vi "File_Driver.vi"(0 "File_Path":path, 2 "Section":string, 5 "Data_In":string, 7 "Key":string, 11 "Error_In":errorcluster, 13 "File_Operation_Select":T1=enum."Close") -> (6 "Data_Out":string, 15 "Error_Out":errorcluster)   [LabVIEW 2021]
uses:
  <vilib>/Utility/config.llb/NI_LVConfig.lvlib
  <vilib>/Utility/config.llb/Read Key (String).vi
  <vilib>/Utility/config.llb/Config Data RefNum.ctl
  <vilib>/Utility/config.llb/Write Key (String).vi
  Controls/File_Operation_Select.ctl
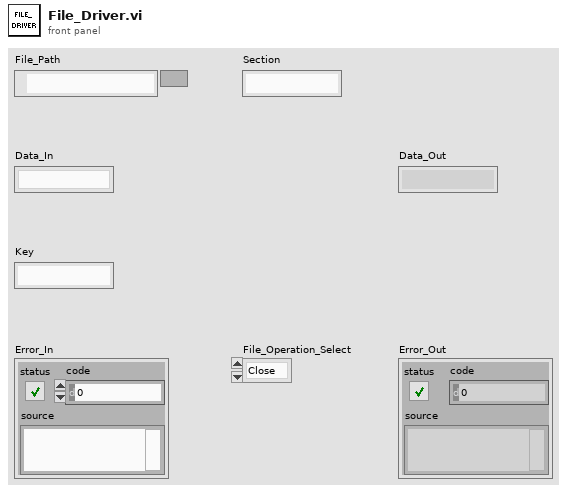
[diagram p1: front panel]
types:
  T1 = typedef "File_Operation_Select.ctl" = enum16{"Open", "Read", "Write", "Close"}
  T2 = typedef "NI_LVConfig.lvlib/Config Data RefNum.ctl" = refnum<k1>
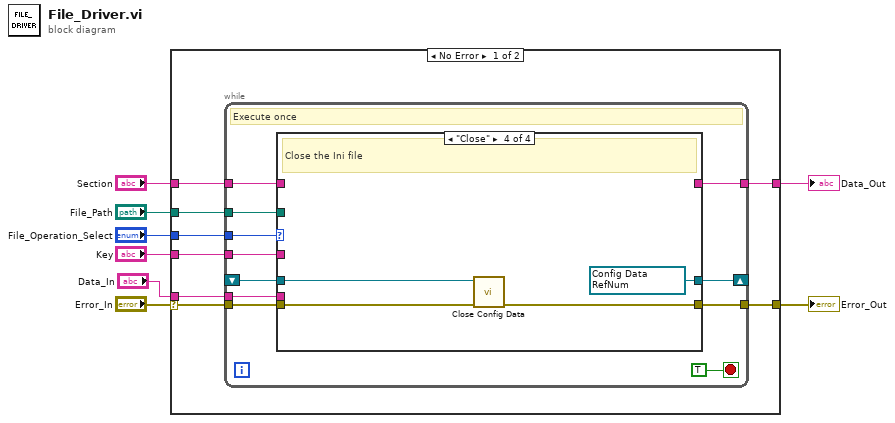
[diagram p0: block diagram]
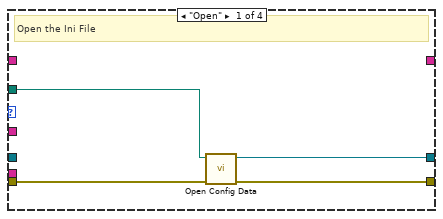
[diagram p2: hidden frame]
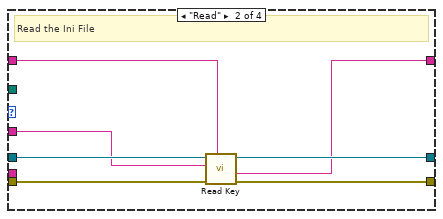
[diagram p3: hidden frame]
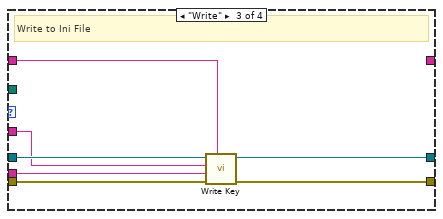
[diagram p4: hidden frame]
diagram:
  n1 = case shown="No Error" "Error_In" {
    selector: "Error_In" -> [w10 w50]
    tunnel: [w16 w50] -> w8
    tunnel: "File_Operation_Select" -> [w15 _]
    tunnel: "File_Path" -> [w14 _]
    tunnel: "Section" -> [w13 _]
    tunnel: "Key" -> [w12 _]
    tunnel: [w11 _] -> w3
    tunnel: "Data_In" -> [w9 _]
    frame No Error {
      n2 = while {
        tunnel: w10 -> [w27]
        tunnel: [w26] -> w16
        tunnel: w15 -> [w25]
        tunnel: w14 -> [w24]
        shift-right: [w23] -> _
        shift-left: _ -> [w22]
        tunnel: w13 -> [w21]
        tunnel: w12 -> [w20]
        tunnel: [w19] -> w11
        tunnel: w9 -> [w17]
        stop <- TRUE stop-if-true
        # "Execute once"
        n3 = case shown="\"Close\"" w25 {
          tunnel: w27 -> [w31 w38 w45 w49]
          tunnel: [w30 w37 w44 w48] -> w26
          tunnel: w24 -> [w29 _ _ _]
          tunnel: [w28 w35 w43 w46] -> w23
          tunnel: w22 -> [_ w36 w42 w47]
          tunnel: w21 -> [_ w34 w41 _]
          tunnel: w20 -> [_ w33 w40 _]
          tunnel: [_ w32 _ _] -> w19
          tunnel: w17 -> [_ _ w39 _]
          frame "Open" {
            # "Open the Ini File"
            n4 = call <vilib>:"Open Config Data.vi"("error in (no error)"=w31, "configuration file path"=w29) -> ("error out"=w30:errorcluster, "refnum"=w28:T2)  [unwired: 7 in, 1 out]
          }
          frame "Read" {
            # "Read the Ini File"
            n5 = call-poly <vilib>:"Read Key.vi"("section"=w34, "error in (no error)"=w38, "key"=w33, "refnum"=w36) -> ("error out"=w37:errorcluster, "value"=w32:string, "refnum out"=w35:T2)  [unwired: 4 in, 1 out]
          }
          frame "Write" {
            # "Write to Ini File"
            n6 = call-poly <vilib>:"Write Key.vi"("section"=w41, "error in (no error)"=w45, "value"=w39, "key"=w40, "refnum"=w42) -> ("error out"=w44:errorcluster, "refnum out"=w43:T2)  [unwired: 4 in, 1 out]
          }
          frame "Close" {
            w46 = T2 refnum items=["config data"] ("refnum out")
            # "Close the Ini file"
            n7 = call <vilib>:"Close Config Data.vi"("error in (no error)"=w49, "refnum"=w47) -> ("error out"=w48:errorcluster)  [unwired: 8 in, 1 out]
          }
        }
      }
    }
    frame Error {
    }
  }
  "Error_Out" <- w8
  "Data_Out" <- w3
